vi "Fetch Room Size Details.vi"(0 "Central Data Manager in":refnum<class "Central Data Manager.lvclass">, 5 "Room No":string, 11 "error in (no error)":errorcluster) -> (4 "Central Data Manager out":refnum<class "Central Data Manager.lvclass">, 6 "Room Size Details":T1, 15 "error out":errorcluster)   [LabVIEW 2023, in "Central Data Manager.lvlib" / "Central Data Manager.lvclass"]
uses:
  Central Data Manager.lvclass
  Central Data Manager.lvclass/Central Data Manager.ctl
  Room Size Details.ctl
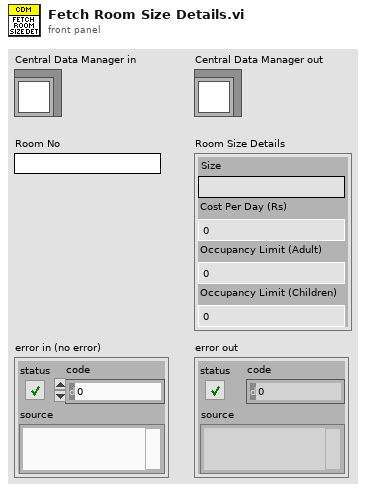
[diagram p1: front panel]
types:
  T1 = typedef "Central Data Manager.lvlib/Central Data Manager.lvclass/Room Size Details.ctl" = cluster{"Size":string, "Cost Per Day (Rs)":u32, "Occupancy Limit (Adult)":u32, "Occupancy Limit (Children)":u32}
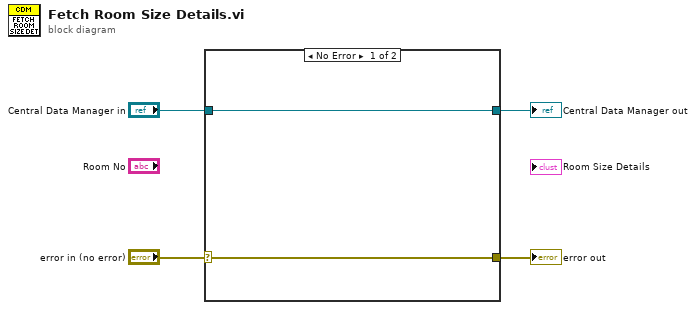
[diagram p0: block diagram]
diagram:
  n1 = case shown="No Error" "error in (no error)" {
    selector: "error in (no error)" -> [w6 w7]
    tunnel: [w6 w7] -> w3
    tunnel: "Central Data Manager in" -> [w5 w8]
    tunnel: [w5 w8] -> w1
    frame No Error {
    }
    frame Error {
    }
  }
  "error out" <- w3
  "Central Data Manager out" <- w1
